vi "Initialize.vi"(8 "error in (no error)":errorcluster caption="错误输入（无错误）", 10 "多功能源VISA":refnum<visa-resource-name>, 11 "5720A 输入":refnum<class "5720A.lvclass">) -> (0 "error out":errorcluster caption="错误输出", 3 "5720A 输出":refnum<class "5720A.lvclass">)   [LabVIEW 2020, in "5720A.lvlib" / "5720A.lvclass"]
uses:
  5720A.lvclass
  <instrlib>/Fluke 5XXX Series Multicalibrators/Fluke 5XXX Series Multicalibrators.lvlib
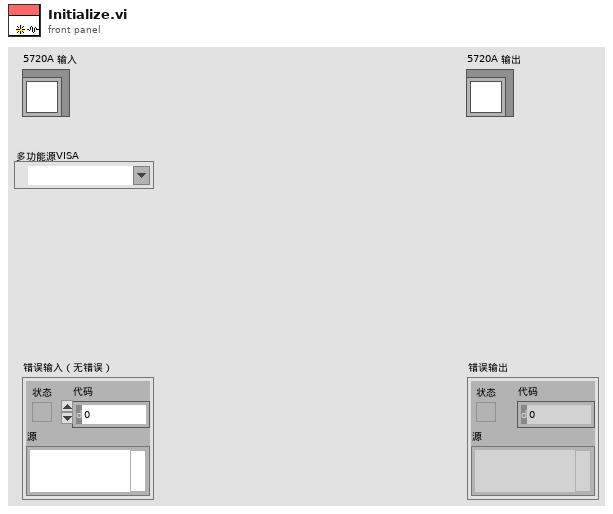
[diagram p1: front panel]
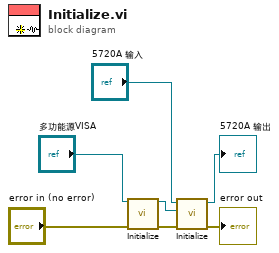
[diagram p0: block diagram]
diagram:
  n1 = call <instrlib>:"Initialize.vi"("VISA resource name"="多功能源VISA", "error in (no error)"="error in (no error)") -> ("VISA resource name out"=w3:refnum<visa-resource-name>, "error out"=w2:errorcluster)  [unwired: 12 in]
  n2 = call-parent <instrlib>:"Initialize.vi"("error in (no error)"=w2, "多功能源VISA"=w3, "多功能校准源接口 输入"="5720A 输入") -> ("error out"=→"error out":errorcluster, "多功能校准源接口 输出"=→"5720A 输出":refnum<class "5720A.lvclass">)  [unwired: 7 in]
